vi "Trigger Settings.vi"(8 "error in (no error)":errorcluster, 11 "Orca-Flash 4.0 in":refnum<class "Orca-Flash 4.0 V2.lvclass">) -> (0 "error out":errorcluster, 3 "Orca-Flash 4.0 out":refnum<class "Orca-Flash 4.0 V2.lvclass">)   [LabVIEW 2018, in "Orca-Flash 4.0 V2.lvlib" / "Orca-Flash 4.0 V2.lvclass"]
uses:
  Orca-Flash 4.0 V2.lvclass
  Orca-Flash 4.0 V2.lvclass/Orca-Flash 4.0 V2.ctl
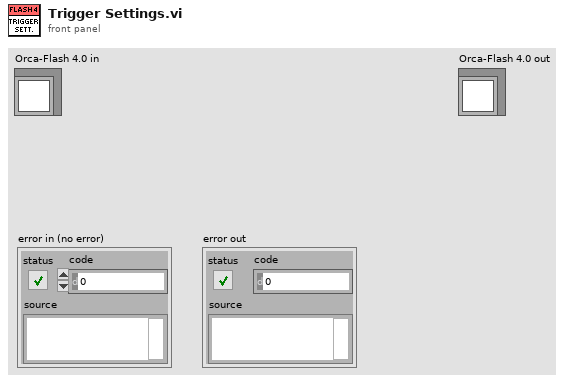
[diagram p1: front panel]
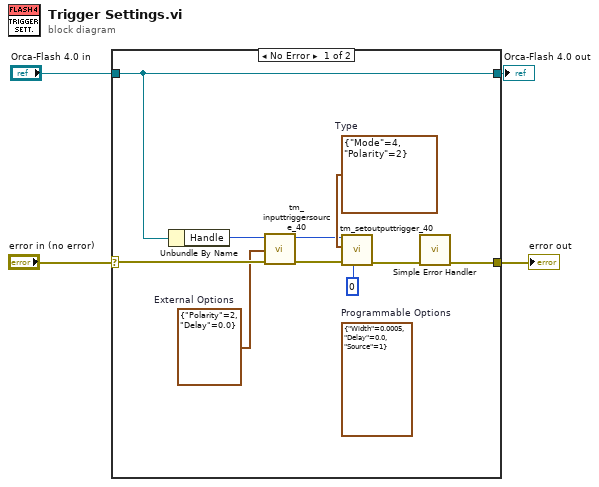
[diagram p0: block diagram]
diagram:
  n1 = case shown="No Error" "error in (no error)" {
    selector: "error in (no error)" -> [w10 w16]
    tunnel: [w5 w16] -> w3
    tunnel: "Orca-Flash 4.0 in" -> [w14 w15]
    tunnel: [w14 w15] -> w1
    frame No Error {
      w7 = cluster{"Polarity":i32, "Delay":dbl} {"Polarity"=2, "Delay"=0.0}  # External Options
      w13 = cluster{"Mode":u32, "Polarity":u32} {"Mode"=4, "Polarity"=2}  # Type
      (unwired) cluster{"Width":dbl, "Delay":dbl, "Source":u32} {"Width"=0.0005, "Delay"=0.0, "Source"=1}  # Programmable Options
      n2 = Unbundle By Name(w14) -> ("Handle"=w8:u32)
      n3 = call <userlib>:"tm_inputtriggersource_40.vi"("error in (no error)"=w10, "External Options"=w7, "Handle in"=w8) -> ("error out"=w11:errorcluster, "Handle out"=w9:u32)  [unwired: 7 in]
      n4 = call <userlib>:"tm_setoutputtrigger_40.vi"("Port"=0, "error in (no error)"=w11, "Type"=w13, "Handle in"=w9) -> ("error out"=w6:errorcluster)  [unwired: 6 in, 1 out]
      n5 = call <vilib>:"Simple Error Handler.vi"("error in (no error)"=w6) -> ("error out"=w5:errorcluster)  [unwired: 4 in, 4 out]
    }
    frame Error {
    }
  }
  "error out" <- w3
  "Orca-Flash 4.0 out" <- w1
